vi "Main_Force_Evaluation.vi"(0 "VISA Refnum in":refnum<visa-resource-name>, 5 "Positions to reach":dbl[](array[numeric]), 7 "Store cluster position":cluster{"Load":dbl}, 9 "Store cluster current":cluster{"Load":dbl}, 11 "error in (no error)":errorcluster) -> (3 "Current (mA)":dbl[](array[numeric]), 4 "VISA Refnum out":refnum<visa-resource-name>, 6 "Actual positions":dbl[](array[numeric]), 8 "New positions to reach":dbl[](array[numeric]), 13 "Positions to Excel":T1, 14 "Currents to Excel":T1, 15 "error out":errorcluster)   [LabVIEW 2015]
uses:
  <vilib>/silver_ctls/ArrayMatrixCluster/Real Matrix NI_Silver.ctl
  <instrlib>/Dynamixel Motor/Dynamixel Motor.lvlib
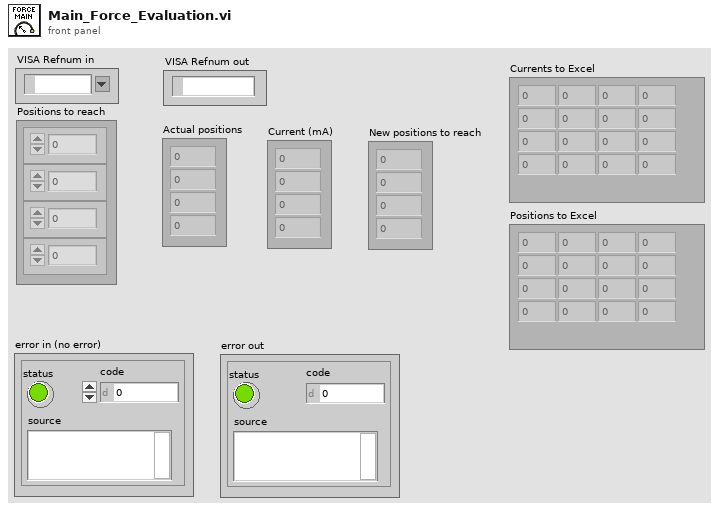
[diagram p1: front panel]
types:
  T1 = typedef "Real Matrix NI_Silver.ctl" = dbl[][]
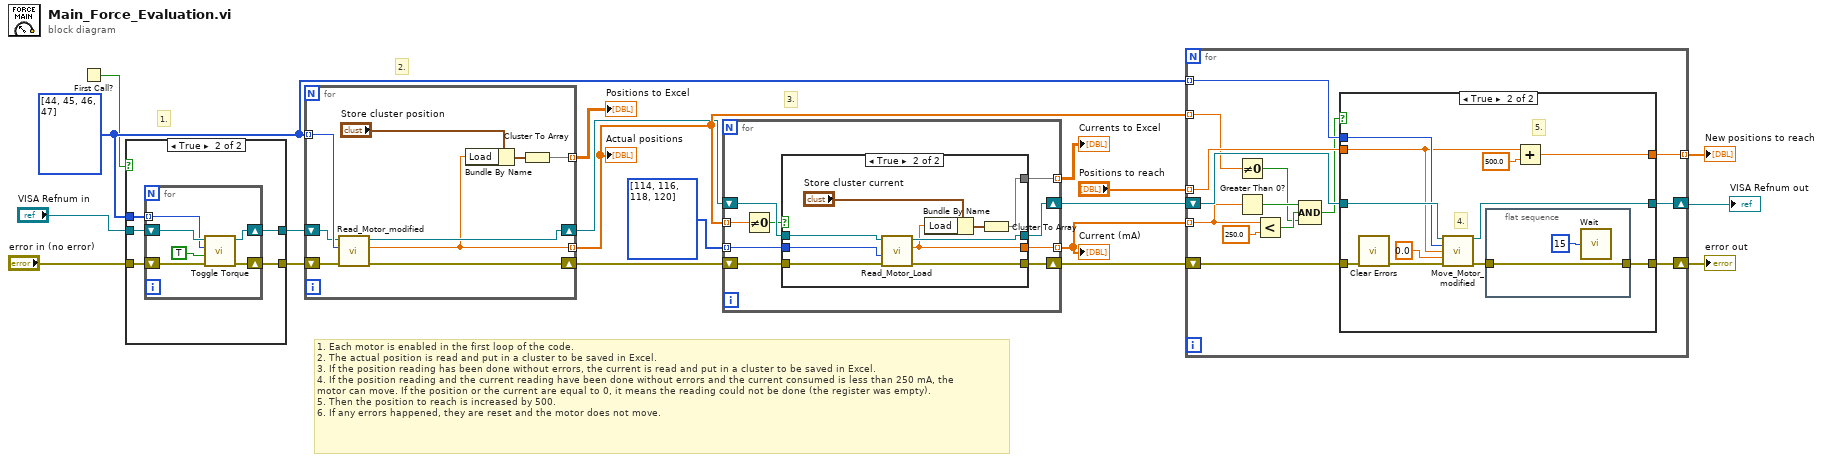
[diagram p0: block diagram]
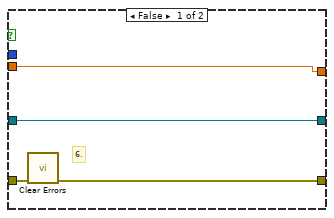
[diagram p2: hidden frame]
diagram:
  w5 = i32[] [44, 45, 46, 47] ("y")
  # "3."
  # "2."
  # "1."
  # "1. Each motor is enabled in the first loop of the code.\n2. The actual position is read and put in a cluster to be saved in Excel.\n3. If the position reading has been done without errors, the current is read and put in a cluster to be saved in Excel.\n4. If the position reading and the current reading have been done without errors and the current consumed is less than 250 mA, the \nmotor can move. If the position or the current are equal to 0, it means the reading could not be done (the register was empty).\n5. Then the position to reach is increased by 500.\n6. If any errors happened, they are reset and the motor does not move."
  n1 = First Call?() -> (First Call?: T/F=w4:bool)
  n2 = case shown="True" w4 {
    tunnel: "VISA Refnum in" -> [w20 w26]
    tunnel: "error in (no error)" -> [w21 w25]
    tunnel: [w20 w24] -> w9
    tunnel: [w21 w23] -> w10
    tunnel: w5 -> [_ w22]
    frame False {
    }
    frame True {
      n3 = for {
        shift-right: [w30] -> w24
        shift-left: w26 -> [w31]
        shift-right: [w28] -> w23
        shift-left: w25 -> [w29]
        tunnel: w22 -> [w27] mode=indexing
        n4 = call <instrlib>:"Toggle Torque.vi"("error in (no error)"=w29, "Toggle torque (OFF)"=TRUE, "Motor ID (0)"=w27, "VISA resource name"=w31) -> ("error out"=w28:errorcluster, "VISA resource name out"=w30:refnum<visa-resource-name>)  [unwired: 6 in]
      }
    }
  }
  n5 = for {
    tunnel: w5 -> [w41] mode=indexing
    shift-right: [w33] -> w12
    shift-left: w10 -> [w40]
    shift-right: [w38] -> w11
    shift-left: w9 -> [w39]
    tunnel: [w35] -> w16 mode=indexing
    tunnel: [w34] -> w19 mode=indexing
    n6 = call "Read_Motor_modified.vi"("error in (no error)"=w40, "Motor ID (0)"=w41, "VISA Refnum in"=w39) -> ("error out"=w33:errorcluster, "Position"=w35:dbl, "VISA Refnum out"=w38:refnum<visa-resource-name>)  [unwired: 6 in]
    n7 = Bundle By Name(cluster="Store cluster position", "Load"=w35) -> (w37:cluster{"Load":dbl})
    n8 = Cluster To Array(cluster=w37) -> (array=w34:dbl[])
  }
  "Positions to Excel" <- w19
  "Actual positions" <- w16
  n9 = for {
    shift-right: [w49] -> w13
    shift-left: w11 -> [w50]
    shift-right: [w46] -> w14
    shift-left: w12 -> [w48]
    tunnel: [w44] -> w15 mode=indexing
    tunnel: u8[] [114, 116, 118, 120] ("Address # DEC") -> [w47] mode=indexing
    tunnel: [w45] -> w18 mode=indexing
    tunnel: w16 -> [w43] mode=indexing
    n10 = Not Equal To 0?(x=w43) -> (x != 0?=w42:bool)
    n11 = case shown="True" w42 {
      tunnel: w50 -> [w52 w61]
      tunnel: [w52 w60] -> w49
      tunnel: w48 -> [w51 w59]
      tunnel: w47 -> [_ w58]
      tunnel: [w51 w55] -> w46
      tunnel: [_ w57] -> w45
      tunnel: [_ w56] -> w44
      frame False {
      }
      frame True {
        n12 = call "Read_Motor_Load.vi"("error in (no error)"=w59, "Address"=w58, "VISA Refnum in"=w61) -> ("error out"=w55:errorcluster, "Current load"=w56:dbl, "VISA Refnum out"=w60:refnum<visa-resource-name>)  [unwired: 6 in]
        n13 = Bundle By Name(cluster="Store cluster current", "Load"=w56) -> (w54:cluster{"Load":dbl})
        n14 = Cluster To Array(cluster=w54) -> (array=w57:dbl[])
      }
    }
  }
  "Currents to Excel" <- w18
  "Current (mA)" <- w15
  n15 = for {
    shift-right: [w73] -> w1
    shift-left: w13 -> [w75]
    shift-right: [w70] -> w8
    shift-left: w14 -> [w74]
    tunnel: w5 -> [w72] mode=indexing
    tunnel: "Positions to reach" -> [w71] mode=indexing
    tunnel: w15 -> [w69] mode=indexing
    tunnel: w16 -> [w67] mode=indexing
    tunnel: [w62] -> w17 mode=indexing
    n16 = Not Equal To 0?(x=w67) -> (x != 0?=w64:bool)
    n17 = Greater Than 0?(x=w69) -> (x > 0?=w66:bool)
    n18 = Less?(x=w69, y=250.0) -> (x < y?=w65:bool)
    n19 = Compound Arithmetic op=AND(w66, w65, w64) -> (w63:bool)
    n20 = case shown="True" w63 {
      tunnel: w75 -> [w78 w90]
      tunnel: w74 -> [w79 w83]
      tunnel: [w78 w89] -> w73
      tunnel: w72 -> [_ w88]
      tunnel: w71 -> [w77 w86]
      tunnel: [w76 w80] -> w70
      tunnel: [w77 w84] -> w62
      frame False {
        # "6."
        n21 = call <vilib>:"Clear Errors.vi"("error in (no error)"=w79) -> ("error out"=w76:errorcluster)  [unwired: 5 in, 1 out]
      }
      frame True {
        # "5."
        # "4."
        n22 = call <vilib>:"Clear Errors.vi"("error in (no error)"=w83) -> ("error out"=w82:errorcluster)  [unwired: 5 in, 1 out]
        n23 = call "Move_Motor_modified.vi"("VISA Refnum in"=w90, "Motor ID (0)"=w88, "Goal Position (bit)"=w86, "Goal Speed (RPM)"=0.0, "error in (no error)"=w82) -> ("VISA Refnum out"=w89:refnum<visa-resource-name>, "error out"=w81:errorcluster)  [unwired: 9 in]
        n24 = flat-sequence {
          tunnel: [w91] -> w80
          tunnel: w81 -> [w91]
          frame #0 {
            n25 = call "Wait"("Count(mSec)"=u32 15) -> ()  [unwired: 1 out]
          }
        }
        n26 = Add(x=w86, y=500.0) -> (x+y=w84:dbl)
      }
    }
  }
  "New positions to reach" <- w17
  "error out" <- w8
  "VISA Refnum out" <- w1
